vi "I(V)_K6221-K2182a_PK.vi"() -> ()   [LabVIEW 2016]
uses:
  Labview Drivers/Keithley 622x LV 2009/Keithley 622x.lvlib
panel:
  out "Resistance (ohm)":dbl=inf format="%#_13g"
  out "Time (s)":dbl=183.05660459992941 format="%#_13g"
  in  "Total number of I-V loops":i32=1
  in  "Numeric Average":i32=1
  in  "wait (ms)":u32=50
  out "Iset (A)":dbl
  out "Vmeas (V)":dbl=5.23101808e-07
  in  "Folder":path=path "D:/Pranava/Data/PtTe2/31-05-2022/001/Round8_IP/after warmup"
  in  "Set Compliance voltage (V)":dbl=2.0 min=0.0 step=0.1 format="%_3f"
  out "I vs V":cluster{dbl, "Field Reading":dbl}[](graph)=[{0.0, "Field Reading"=-1.0306718e-07}, {1e-07, "Field Reading"=-6.16332151e-08}, {2e-07, "Field Reading"=7.87243392e-08}, {3e-07, "Field Reading"=1.57966796e-07}, {4e-07, "Field Reading"=4.14402344e-09}, {5e-07, "Field Reading"=-1.72986197e-07}, {6e-07, "Field Reading"=6.26695055e-08}, {7e-07, "Field Reading"=8.13147919e-08}, {8e-07, "Field Reading"=1.95776133e-07}, {9e-07, "Field Reading"=1.06693098e-07}, {1e-06, "Field Reading"=1.80756319e-07}, {1.1e-06, "Field Reading"=-4.14238014e-09}, {1.2e-06, "Field Reading"=-1.20157502e-07}, {1.3e-06, "Field Reading"=1.29491334e-08}, {1.4e-06, "Field Reading"=1.86453892e-07}, {1.5e-06, "Field Reading"=9.68529269e-08}, {1.6e-06, "Field Reading"=-7.61339067e-08}, {1.7e-06, "Field Reading"=2.95227222e-08}, {1.8e-06, "Field Reading"=-1.09281084e-07}, {1.9e-06, "Field Reading"=4.60959452e-08}, {2e-06, "Field Reading"=2.19600694e-07}, {2.1e-06, "Field Reading"=-3.47002959e-08}, {2.2e-06, "Field Reading"=-7.2502909e-09}, {2.3e-06, "Field Reading"=-1.22747482e-07}, {2.4e-06, "Field Reading"=1.51234644e-07}, {2.5e-06, "Field Reading"=2.13903523e-07}, {2.6e-06, "Field Reading"=-1.10320173e-07}, {2.7e-06, "Field Reading"=-9.78899879e-08}, {2.8e-06, "Field Reading"=3.57345042e-08}, {2.9e-06, "Field Reading"=1.22745801e-07}, {3e-06, "Field Reading"=1.53821265e-07}, {3.1e-06, "Field Reading"=5.17696534e-09}, {3.2e-06, "Field Reading"=1.97326913e-07}, {3.3e-06, "Field Reading"=-6.94037265e-08}, {3.4e-06, "Field Reading"=-1.25857489e-07}, {3.5e-06, "Field Reading"=1.51750002e-07}, {3.6e-06, "Field Reading"=2.50673566e-07}, {3.7e-06, "Field Reading"=7.6133036e-08}, {3.8e-06, "Field Reading"=-1.42948994e-07}, {3.9e-06, "Field Reading"=7.76701235e-09}, {4e-06, "Field Reading"=1.305151e-07}, {4.1e-06, "Field Reading"=1.63142241e-07}, {4.2e-06, "Field Reading"=3.10364491e-09}, {4.3e-06, "Field Reading"=-6.21899174e-09}, {4.4e-06, "Field Reading"=3.21074034e-08}, {4.5e-06, "Field Reading"=6.72911471e-09}, {4.6e-06, "Field Reading"=2.5374388e-08}, {4.7e-06, "Field Reading"=7.04337985e-08}, {4.8e-06, "Field Reading"=-8.80770635e-09}, {4.9e-06, "Field Reading"=-1.24331767e-08}, {5e-06, "Field Reading"=-1.79722736e-07}, {5.1e-06, "Field Reading"=7.66498082e-08}, {5.2e-06, "Field Reading"=1.81270523e-07}, {5.3e-06, "Field Reading"=1.70885102e-08}, {5.4e-06, "Field Reading"=-5.54208961e-08}, {5.5e-06, "Field Reading"=-5.38662375e-08}, {5.6e-06, "Field Reading"=1.13922372e-08}, {5.7e-06, "Field Reading"=9.58139147e-08}, {5.8e-06, "Field Reading"=1.48124279e-07}, {5.9e-06, "Field Reading"=1.15495042e-07}, {6e-06, "Field Reading"=-1.23786032e-07}, {6.1e-06, "Field Reading"=2.2786574e-08}, {6.2e-06, "Field Reading"=1.53821448e-07}, {6.3e-06, "Field Reading"=9.21858153e-08}, {6.4e-06, "Field Reading"=1.43978235e-07}, {6.5e-06, "Field Reading"=1.76047313e-08}, {6.6e-06, "Field Reading"=1.2118957e-07}, {6.7e-06, "Field Reading"=5.48952733e-08}, {6.8e-06, "Field Reading"=2.49634771e-07}, {6.9e-06, "Field Reading"=1.08241465e-07}, {7e-06, "Field Reading"=1.1445703e-07}, {7.1e-06, "Field Reading"=-4.29919365e-08}, {7.2e-06, "Field Reading"=-6.73724028e-09}, {7.3e-06, "Field Reading"=-1.37772071e-07}, {7.4e-06, "Field Reading"=5.59315918e-08}, {7.5e-06, "Field Reading"=-5.18346759e-09}, {7.6e-06, "Field Reading"=1.19080321e-08}, {7.7e-06, "Field Reading"=9.37431805e-08}, {7.8e-06, "Field Reading"=-3.10869695e-09}, {7.9e-06, "Field Reading"=1.55894118e-07}, {8e-06, "Field Reading"=1.97846001e-07}, {8.1e-06, "Field Reading"=-7.2510577e-08}, {8.2e-06, "Field Reading"=2.01979046e-08}, {8.3e-06, "Field Reading"=1.89041284e-07}, {8.4e-06, "Field Reading"=2.00953547e-07}, {8.5e-06, "Field Reading"=1.25336495e-07}, {8.6e-06, "Field Reading"=-2.95229225e-08}, {8.7e-06, "Field Reading"=-3.21125449e-08}, {8.8e-06, "Field Reading"=1.46053473e-07}, {8.9e-06, "Field Reading"=4.81657483e-08}, {9e-06, "Field Reading"=3.2629119e-07}, {9.1e-06, "Field Reading"=-2.22719799e-08}, {9.2e-06, "Field Reading"=-3.36631723e-08}, {9.3e-06, "Field Reading"=4.14533263e-09}, {9.4e-06, "Field Reading"=1.62630298e-07}, {9.5e-06, "Field Reading"=2.13904846e-07}, {9.6e-06, "Field Reading"=1.09284052e-07}, {9.7e-06, "Field Reading"=7.19934716e-08}, {9.8e-06, "Field Reading"=3.05594936e-08}, {9.9e-06, "Field Reading"=3.41826524e-08}, {1e-05, "Field Reading"=2.29958129e-07}, {1.01e-05, "Field Reading"=1.10835484e-07}, {1.02e-05, "Field Reading"=5.74892568e-08}, {1.03e-05, "Field Reading"=-1.50198484e-07}, {1.04e-05, "Field Reading"=1.27926994e-07}, {1.05e-05, "Field Reading"=6.21505776e-08}, {1.06e-05, "Field Reading"=2.04579826e-07}, {1.07e-05, "Field Reading"=7.97590954e-08}, {1.08e-05, "Field Reading"=8.75279624e-08}, {1.09e-05, "Field Reading"=1.05137394e-07}, {1.1e-05, "Field Reading"=9.83929215e-09}, {1.11e-05, "Field Reading"=2.01471345e-07}, {1.12e-05, "Field Reading"=1.77128895e-07}, {1.13e-05, "Field Reading"=3.625344e-08}, {1.14e-05, "Field Reading"=-7.92397757e-08}, {1.15e-05, "Field Reading"=1.2585844e-07}, {1.16e-05, "Field Reading"=1.28965989e-07}, {1.17e-05, "Field Reading"=2.76056628e-07}, {1.18e-05, "Field Reading"=1.09284847e-07}, {1.19e-05, "Field Reading"=-1.65708764e-08}, {1.2e-05, "Field Reading"=7.87272845e-08}, {1.21e-05, "Field Reading"=1.05140243e-07}, {1.22e-05, "Field Reading"=2.38246889e-07}, {1.23e-05, "Field Reading"=1.02032695e-07}, {1.24e-05, "Field Reading"=5.80090957e-08}, {1.25e-05, "Field Reading"=1.11355339e-07}, {1.26e-05, "Field Reading"=1.65737432e-07}, {1.27e-05, "Field Reading"=1.9422329e-07}, {1.28e-05, "Field Reading"=2.24780847e-07}, {1.29e-05, "Field Reading"=1.08819028e-08}, {1.3e-05, "Field Reading"=1.2327163e-07}, {1.31e-05, "Field Reading"=7.45866788e-08}, {1.32e-05, "Field Reading"=2.26607776e-05}, {1.33e-05, "Field Reading"=2.30844403e-05}, {1.34e-05, "Field Reading"=2.30253968e-05}, {1.35e-05, "Field Reading"=2.31046393e-05}, {1.36e-05, "Field Reading"=2.33547805e-05}, {1.37e-05, "Field Reading"=2.36748579e-05}, {1.38e-05, "Field Reading"=2.39084419e-05}, {1.39e-05, "Field Reading"=2.39172467e-05}, {1.4e-05, "Field Reading"=2.41093967e-05}, {1.41e-05, "Field Reading"=2.42000335e-05}, {1.42e-05, "Field Reading"=2.44129006e-05}, {1.43e-05, "Field Reading"=2.46739283e-05}, {1.44e-05, "Field Reading"=2.49126915e-05}, {1.45e-05, "Field Reading"=2.50665151e-05}, {1.46e-05, "Field Reading"=2.49173528e-05}, {1.47e-05, "Field Reading"=2.53726085e-05}, {1.48e-05, "Field Reading"=2.56072284e-05}, {1.49e-05, "Field Reading"=2.57211718e-05}, {1.5e-05, "Field Reading"=2.58874256e-05}, {1.51e-05, "Field Reading"=2.59397274e-05}, {1.52e-05, "Field Reading"=2.62603227e-05}, {1.53e-05, "Field Reading"=2.64281302e-05}, {1.54e-05, "Field Reading"=2.65425915e-05}, {1.55e-05, "Field Reading"=2.69118716e-05}, {1.56e-05, "Field Reading"=2.69351782e-05}, {1.57e-05, "Field Reading"=2.69346603e-05}, {1.58e-05, "Field Reading"=2.71889769e-05}, {1.59e-05, "Field Reading"=2.76551091e-05}, {1.6e-05, "Field Reading"=2.7724511e-05}, {1.61e-05, "Field Reading"=2.77509251e-05}, {1.62e-05, "Field Reading"=2.79042308e-05}, {1.63e-05, "Field Reading"=2.81564602e-05}, {1.64e-05, "Field Reading"=2.83128734e-05}, {1.65e-05, "Field Reading"=2.85402591e-05}, {1.66e-05, "Field Reading"=2.878213e-05}, {1.67e-05, "Field Reading"=2.86754375e-05}, {1.68e-05, "Field Reading"=2.90255548e-05}, {1.69e-05, "Field Reading"=2.92524059e-05}, {1.7e-05, "Field Reading"=2.948599e-05}, {1.71e-05, "Field Reading"=2.95517665e-05}, {1.72e-05, "Field Reading"=2.96398137e-05}, {1.73e-05, "Field Reading"=2.98386812e-05}, {1.74e-05, "Field Reading"=2.99769671e-05}, {1.75e-05, "Field Reading"=3.02333399e-05}, {1.76e-05, "Field Reading"=3.06248909e-05}, {1.77e-05, "Field Reading"=3.07186353e-05}, {1.78e-05, "Field Reading"=3.0720707e-05}, {1.79e-05, "Field Reading"=3.07781966e-05}, {1.8e-05, "Field Reading"=3.11676923e-05}, {1.81e-05, "Field Reading"=3.14023123e-05}, {1.82e-05, "Field Reading"=3.14753397e-05}, {1.83e-05, "Field Reading"=3.14453001e-05}, {1.84e-05, "Field Reading"=3.17555371e-05}, {1.85e-05, "Field Reading"=3.203936e-05}, {1.86e-05, "Field Reading"=3.2266729e-05}, {1.87e-05, "Field Reading"=3.2533957e-05}, {1.88e-05, "Field Reading"=3.24930409e-05}, {1.89e-05, "Field Reading"=3.25805702e-05}, {1.9e-05, "Field Reading"=3.27084976e-05}, {1.91e-05, "Field Reading"=3.31010845e-05}, {1.92e-05, "Field Reading"=3.33186128e-05}, {1.93e-05, "Field Reading"=3.33092902e-05}, {1.94e-05, "Field Reading"=3.35133525e-05}, {1.95e-05, "Field Reading"=3.36200314e-05}, {1.96e-05, "Field Reading"=3.38396313e-05}, {1.97e-05, "Field Reading"=3.42684728e-05}, {1.98e-05, "Field Reading"=3.43093888e-05}, {1.99e-05, "Field Reading"=3.4376719e-05}, {2e-05, "Field Reading"=3.4630502e-05}, {2.01e-05, "Field Reading"=3.48371538e-05}, {2.02e-05, "Field Reading"=3.50759123e-05}, {2.03e-05, "Field Reading"=3.52696161e-05}, {2.04e-05, "Field Reading"=3.52986198e-05}, {2.05e-05, "Field Reading"=3.54146349e-05}, {2.06e-05, "Field Reading"=3.56922424e-05}, {2.07e-05, "Field Reading"=3.58439942e-05}, {2.08e-05, "Field Reading"=3.61733941e-05}, {2.09e-05, "Field Reading"=3.62407028e-05}, {2.1e-05, "Field Reading"=3.63385905e-05}, {2.11e-05, "Field Reading"=3.65343658e-05}, {2.12e-05, "Field Reading"=3.68093835e-05}, {2.13e-05, "Field Reading"=3.70973494e-05}, {2.14e-05, "Field Reading"=3.70709352e-05}, {2.15e-05, "Field Reading"=3.72884634e-05}, {2.16e-05, "Field Reading"=3.74443585e-05}, {2.17e-05, "Field Reading"=3.75831529e-05}, {2.18e-05, "Field Reading"=3.7787215e-05}, {2.19e-05, "Field Reading"=3.808036e-05}, {2.2e-05, "Field Reading"=3.80984874e-05}, {2.21e-05, "Field Reading"=3.8141475e-05}, {2.22e-05, "Field Reading"=3.84734643e-05}, {2.23e-05, "Field Reading"=3.87127452e-05}, {2.24e-05, "Field Reading"=3.88867762e-05}, {2.25e-05, "Field Reading"=3.90576911e-05}, {2.26e-05, "Field Reading"=3.91959769e-05}, {2.27e-05, "Field Reading"=3.9318207e-05}, {2.28e-05, "Field Reading"=3.95512728e-05}, {2.29e-05, "Field Reading"=3.98946565e-05}, {2.3e-05, "Field Reading"=4.00065281e-05}, {2.31e-05, "Field Reading"=4.00277984e-05}, {2.32e-05, "Field Reading"=4.02308248e-05}, {2.33e-05, "Field Reading"=4.04452456e-05}, {2.34e-05, "Field Reading"=4.06151248e-05}, {2.35e-05, "Field Reading"=4.08015776e-05}, {2.36e-05, "Field Reading"=4.10191059e-05}, {2.37e-05, "Field Reading"=4.11428899e-05}, {2.38e-05, "Field Reading"=4.12573512e-05}, {2.39e-05, "Field Reading"=4.1494075e-05}, {2.4e-05, "Field Reading"=4.17799696e-05}, {2.41e-05, "Field Reading"=4.19229168e-05}, {2.42e-05, "Field Reading"=4.19032357e-05}, {2.43e-05, "Field Reading"=4.21290509e-05}, {2.44e-05, "Field Reading"=4.22953048e-05}, {2.45e-05, "Field Reading"=4.26832305e-05}, {2.46e-05, "Field Reading"=4.28903968e-05}, {2.47e-05, "Field Reading"=4.29478865e-05}, {2.48e-05, "Field Reading"=4.30939413e-05}, {2.49e-05, "Field Reading"=4.32783225e-05}, {2.5e-05, "Field Reading"=4.35756113e-05}, {2.51e-05, "Field Reading"=4.37413473e-05}, {2.52e-05, "Field Reading"=4.394282e-05}, {2.53e-05, "Field Reading"=4.40370823e-05}, {2.54e-05, "Field Reading"=4.41116635e-05}, {2.55e-05, "Field Reading"=4.42986344e-05}, {2.56e-05, "Field Reading"=4.46016204e-05}, {2.57e-05, "Field Reading"=4.49289489e-05}, {2.58e-05, "Field Reading"=4.4907196e-05}, {2.59e-05, "Field Reading"=4.49828131e-05}, {2.6e-05, "Field Reading"=4.51438877e-05}, {2.61e-05, "Field Reading"=4.53893525e-05}, {2.62e-05, "Field Reading"=4.57192705e-05}, {2.63e-05, "Field Reading"=4.58549667e-05}, {2.64e-05, "Field Reading"=4.59787506e-05}, {2.65e-05, "Field Reading"=4.61569167e-05}, {2.66e-05, "Field Reading"=4.6195761e-05}, {2.67e-05, "Field Reading"=4.65381091e-05}, {2.68e-05, "Field Reading"=4.68421046e-05}, {2.69e-05, "Field Reading"=4.69166857e-05}, {2.7e-05, "Field Reading"=4.69291159e-05}, {2.71e-05, "Field Reading"=4.70637762e-05}, {2.72e-05, "Field Reading"=4.74589524e-05}, {2.73e-05, "Field Reading"=4.76852853e-05}, {2.74e-05, "Field Reading"=4.7755723e-05}, {2.75e-05, "Field Reading"=4.79189044e-05}, {2.76e-05, "Field Reading"=4.80960347e-05}, {2.77e-05, "Field Reading"=4.8176313e-05}, {2.78e-05, "Field Reading"=4.85476649e-05}, {2.79e-05, "Field Reading"=4.87708904e-05}, {2.8e-05, "Field Reading"=4.86621262e-05}, {2.81e-05, "Field Reading"=4.89531998e-05}, {2.82e-05, "Field Reading"=4.91298121e-05}, {2.83e-05, "Field Reading"=4.93898453e-05}, {2.84e-05, "Field Reading"=4.9613071e-05}, {2.85e-05, "Field Reading"=4.97399626e-05}, {2.86e-05, "Field Reading"=4.98943042e-05}, {2.87e-05, "Field Reading"=4.98109183e-05}, {2.88e-05, "Field Reading"=5.01926289e-05}, {2.89e-05, "Field Reading"=5.05764113e-05}, {2.9e-05, "Field Reading"=5.06804975e-05}, {2.91e-05, "Field Reading"=5.06680673e-05}, {2.92e-05, "Field Reading"=5.07587041e-05}, {2.93e-05, "Field Reading"=5.11942789e-05}, {2.94e-05, "Field Reading"=5.126886e-05}, {2.95e-05, "Field Reading"=5.15138384e-05}, {2.96e-05, "Field Reading"=5.16236385e-05}, {2.97e-05, "Field Reading"=5.17816017e-05}, {2.98e-05, "Field Reading"=5.19965405e-05}, {2.99e-05, "Field Reading"=5.21840292e-05}, {3e-05, "Field Reading"=5.24512784e-05}, {3e-05, "Field Reading"=5.23492472e-05}, {2.99e-05, "Field Reading"=5.22622359e-05}, {2.98e-05, "Field Reading"=5.19255848e-05}, {2.97e-05, "Field Reading"=5.18157848e-05}, {2.96e-05, "Field Reading"=5.18442655e-05}, {2.95e-05, "Field Reading"=5.17018363e-05}, {2.94e-05, "Field Reading"=5.13310022e-05}, {2.93e-05, "Field Reading"=5.10901672e-05}, {2.92e-05, "Field Reading"=5.09461842e-05}, {2.91e-05, "Field Reading"=5.08710851e-05}, {2.9e-05, "Field Reading"=5.07504086e-05}, {2.89e-05, "Field Reading"=5.04069981e-05}, {2.88e-05, "Field Reading"=5.03842094e-05}, {2.87e-05, "Field Reading"=5.00076783e-05}, {2.86e-05, "Field Reading"=4.98393529e-05}, {2.85e-05, "Field Reading"=4.98072416e-05}, {2.84e-05, "Field Reading"=4.97787557e-05}, {2.83e-05, "Field Reading"=4.92551341e-05}, {2.82e-05, "Field Reading"=4.91329288e-05}, {2.81e-05, "Field Reading"=4.90909769e-05}, {2.8e-05, "Field Reading"=4.89148825e-05}, {2.79e-05, "Field Reading"=4.88750023e-05}, {2.78e-05, "Field Reading"=4.85186701e-05}, {2.77e-05, "Field Reading"=4.84611805e-05}, {2.76e-05, "Field Reading"=4.79670804e-05}, {2.75e-05, "Field Reading"=4.794222e-05}, {2.74e-05, "Field Reading"=4.79997168e-05}, {2.73e-05, "Field Reading"=4.7894578e-05}, {2.72e-05, "Field Reading"=4.74450194e-05}, {2.71e-05, "Field Reading"=4.71798419e-05}, {2.7e-05, "Field Reading"=4.71342645e-05}, {2.69e-05, "Field Reading"=4.70327513e-05}, {2.68e-05, "Field Reading"=4.68369757e-05}, {2.67e-05, "Field Reading"=4.66453199e-05}, {2.66e-05, "Field Reading"=4.64552416e-05}, {2.65e-05, "Field Reading"=4.61289491e-05}, {2.64e-05, "Field Reading"=4.60574756e-05}, {2.63e-05, "Field Reading"=4.59326557e-05}, {2.62e-05, "Field Reading"=4.57897086e-05}, {2.61e-05, "Field Reading"=4.55690727e-05}, {2.6e-05, "Field Reading"=4.53670553e-05}, {2.59e-05, "Field Reading"=4.51086111e-05}, {2.58e-05, "Field Reading"=4.51402045e-05}, {2.57e-05, "Field Reading"=4.5013831e-05}, {2.56e-05, "Field Reading"=4.45886152e-05}, {2.55e-05, "Field Reading"=4.43975011e-05}, {2.54e-05, "Field Reading"=4.42659484e-05}, {2.53e-05, "Field Reading"=4.42783786e-05}, {2.52e-05, "Field Reading"=4.4098133e-05}, {2.51e-05, "Field Reading"=4.38241511e-05}, {2.5e-05, "Field Reading"=4.36066229e-05}, {2.49e-05, "Field Reading"=4.35335956e-05}, {2.48e-05, "Field Reading"=4.31845148e-05}, {2.47e-05, "Field Reading"=4.3292243e-05}, {2.46e-05, "Field Reading"=4.31876223e-05}, {2.45e-05, "Field Reading"=4.27178684e-05}, {2.44e-05, "Field Reading"=4.25132884e-05}, {2.43e-05, "Field Reading"=4.23843252e-05}, {2.42e-05, "Field Reading"=4.23439272e-05}, {2.41e-05, "Field Reading"=4.22191074e-05}, {2.4e-05, "Field Reading"=4.20766783e-05}, {2.39e-05, "Field Reading"=4.17011832e-05}, {2.38e-05, "Field Reading"=4.15660192e-05}, {2.37e-05, "Field Reading"=4.13101646e-05}, {2.36e-05, "Field Reading"=4.12019184e-05}, {2.35e-05, "Field Reading"=4.12506033e-05}, {2.34e-05, "Field Reading"=4.08316025e-05}, {2.33e-05, "Field Reading"=4.06140743e-05}, {2.32e-05, "Field Reading"=4.05224017e-05}, {2.31e-05, "Field Reading"=4.03825621e-05}, {2.3e-05, "Field Reading"=4.02712359e-05}, {2.29e-05, "Field Reading"=4.00718349e-05}, {2.28e-05, "Field Reading"=3.96419574e-05}, {2.27e-05, "Field Reading"=3.95616791e-05}, {2.26e-05, "Field Reading"=3.954148e-05}, {2.25e-05, "Field Reading"=3.93596885e-05}, {2.24e-05, "Field Reading"=3.92970196e-05}, {2.23e-05, "Field Reading"=3.89966273e-05}, {2.22e-05, "Field Reading"=3.87247169e-05}, {2.21e-05, "Field Reading"=3.85626064e-05}, {2.2e-05, "Field Reading"=3.85646781e-05}, {2.19e-05, "Field Reading"=3.83637233e-05}, {2.18e-05, "Field Reading"=3.81353185e-05}, {2.17e-05, "Field Reading"=3.7795042e-05}, {2.16e-05, "Field Reading"=3.77416642e-05}, {2.15e-05, "Field Reading"=3.75935378e-05}, {2.14e-05, "Field Reading"=3.74614671e-05}, {2.13e-05, "Field Reading"=3.72662096e-05}, {2.12e-05, "Field Reading"=3.72004332e-05}, {2.11e-05, "Field Reading"=3.67658947e-05}, {2.1e-05, "Field Reading"=3.67462136e-05}, {2.09e-05, "Field Reading"=3.66597202e-05}, {2.08e-05, "Field Reading"=3.65121165e-05}, {2.07e-05, "Field Reading"=3.61992902e-05}, {2.06e-05, "Field Reading"=3.60371798e-05}, {2.05e-05, "Field Reading"=3.58382969e-05}, {2.04e-05, "Field Reading"=3.58035959e-05}, {2.03e-05, "Field Reading"=3.56699714e-05}, {2.02e-05, "Field Reading"=3.53680215e-05}, {2.01e-05, "Field Reading"=3.5284114e-05}, {2e-05, "Field Reading"=3.49588575e-05}, {1.99e-05, "Field Reading"=3.48128029e-05}, {1.98e-05, "Field Reading"=3.46719275e-05}, {1.97e-05, "Field Reading"=3.46382624e-05}, {1.96e-05, "Field Reading"=3.44782238e-05}, {1.95e-05, "Field Reading"=3.40566333e-05}, {1.94e-05, "Field Reading"=3.39380163e-05}, {1.93e-05, "Field Reading"=3.3864471e-05}, {1.92e-05, "Field Reading"=3.37702088e-05}, {1.91e-05, "Field Reading"=3.33993751e-05}, {1.9e-05, "Field Reading"=3.33009695e-05}, {1.89e-05, "Field Reading"=3.31865083e-05}, {1.88e-05, "Field Reading"=3.28483038e-05}, {1.87e-05, "Field Reading"=3.2840017e-05}, {1.86e-05, "Field Reading"=3.2770645e-05}, {1.85e-05, "Field Reading"=3.24774997e-05}, {1.84e-05, "Field Reading"=3.21273827e-05}, {1.83e-05, "Field Reading"=3.198081e-05}, {1.82e-05, "Field Reading"=3.19005317e-05}, {1.81e-05, "Field Reading"=3.19274638e-05}, {1.8e-05, "Field Reading"=3.16332826e-05}, {1.79e-05, "Field Reading"=3.13919284e-05}, {1.78e-05, "Field Reading"=3.12945586e-05}, {1.77e-05, "Field Reading"=3.1037668e-05}, {1.76e-05, "Field Reading"=3.0982768e-05}, {1.75e-05, "Field Reading"=3.07522915e-05}, {1.74e-05, "Field Reading"=3.05114566e-05}, {1.73e-05, "Field Reading"=3.03555613e-05}, {1.72e-05, "Field Reading"=2.9926711e-05}, {1.71e-05, "Field Reading"=2.99919695e-05}, {1.7e-05, "Field Reading"=2.98562733e-05}, {1.69e-05, "Field Reading"=2.97961941e-05}, {1.68e-05, "Field Reading"=2.94077507e-05}, {1.67e-05, "Field Reading"=2.92373536e-05}, {1.66e-05, "Field Reading"=2.89794272e-05}, {1.65e-05, "Field Reading"=2.90410602e-05}, {1.64e-05, "Field Reading"=2.9025534e-05}, {1.63e-05, "Field Reading"=2.8613266e-05}, {1.62e-05, "Field Reading"=2.8304065e-05}, {1.61e-05, "Field Reading"=2.81833885e-05}, {1.6e-05, "Field Reading"=2.82476112e-05}, {1.59e-05, "Field Reading"=2.79477328e-05}, {1.58e-05, "Field Reading"=2.77835507e-05}, {1.57e-05, "Field Reading"=2.76204056e-05}, {1.56e-05, "Field Reading"=2.74230763e-05}, {1.55e-05, "Field Reading"=2.71273413e-05}, {1.54e-05, "Field Reading"=2.70154696e-05}, {1.53e-05, "Field Reading"=2.69175818e-05}, {1.52e-05, "Field Reading"=2.67647941e-05}, {1.51e-05, "Field Reading"=2.65156723e-05}, {1.5e-05, "Field Reading"=2.61707402e-05}, {1.49e-05, "Field Reading"=2.59412995e-05}, {1.48e-05, "Field Reading"=2.62018157e-05}, {1.47e-05, "Field Reading"=2.58382325e-05}, {1.46e-05, "Field Reading"=2.55549277e-05}, {1.45e-05, "Field Reading"=2.53472399e-05}, {1.44e-05, "Field Reading"=2.51789143e-05}, {1.43e-05, "Field Reading"=2.52317427e-05}, {1.42e-05, "Field Reading"=2.49158009e-05}, {1.41e-05, "Field Reading"=2.4860383e-05}, {1.4e-05, "Field Reading"=2.4564648e-05}, {1.39e-05, "Field Reading"=2.44734933e-05}, {1.38e-05, "Field Reading"=2.4090747e-05}, {1.37e-05, "Field Reading"=2.41896706e-05}, {1.36e-05, "Field Reading"=2.40135762e-05}, {1.35e-05, "Field Reading"=2.36494645e-05}, {1.34e-05, "Field Reading"=2.34490277e-05}, {1.33e-05, "Field Reading"=2.34132909e-05}, {1.32e-05, "Field Reading"=2.32630928e-05}, {1.31e-05, "Field Reading"=2.30554051e-05}, {1.3e-05, "Field Reading"=2.2857558e-05}, {1.29e-05, "Field Reading"=2.26534958e-05}, {1.28e-05, "Field Reading"=2.24659978e-05}, {1.27e-05, "Field Reading"=2.21987489e-05}, {1.26e-05, "Field Reading"=2.21935697e-05}, {1.25e-05, "Field Reading"=2.21143273e-05}, {1.24e-05, "Field Reading"=2.17611029e-05}, {1.23e-05, "Field Reading"=2.14622606e-05}, {1.22e-05, "Field Reading"=2.12483579e-05}, {1.21e-05, "Field Reading"=2.13529786e-05}, {1.2e-05, "Field Reading"=2.11416515e-05}, {1.19e-05, "Field Reading"=2.08101801e-05}, {1.18e-05, "Field Reading"=2.06154407e-05}, {1.17e-05, "Field Reading"=2.04750833e-05}, {1.16e-05, "Field Reading"=2.03026146e-05}, {1.15e-05, "Field Reading"=2.02016194e-05}, {1.14e-05, "Field Reading"=2.00322583e-05}, {1.13e-05, "Field Reading"=1.98173324e-05}, {1.12e-05, "Field Reading"=1.95884099e-05}, {1.11e-05, "Field Reading"=1.93770968e-05}, {1.1e-05, "Field Reading"=1.94936298e-05}, {1.09e-05, "Field Reading"=1.92268988e-05}, {1.08e-05, "Field Reading"=1.8910965e-05}, {1.07e-05, "Field Reading"=1.86789349e-05}, {1.06e-05, "Field Reading"=1.83878552e-05}, {1.05e-05, "Field Reading"=1.84510419e-05}, {1.04e-05, "Field Reading"=1.81604865e-05}, {1.03e-05, "Field Reading"=1.80449894e-05}, {1.02e-05, "Field Reading"=1.78657877e-05}, {1.01e-05, "Field Reading"=1.75462285e-05}, {1e-05, "Field Reading"=1.73349154e-05}, {9.9e-06, "Field Reading"=1.73618475e-05}, {9.8e-06, "Field Reading"=1.71360338e-05}, {9.7e-06, "Field Reading"=1.6854801e-05}, {9.6e-06, "Field Reading"=1.65616559e-05}, {9.5e-06, "Field Reading"=1.63736494e-05}, {9.4e-06, "Field Reading"=1.64119758e-05}, {9.3e-06, "Field Reading"=1.62643674e-05}, {9.2e-06, "Field Reading"=1.5946362e-05}, {9.1e-06, "Field Reading"=1.58489938e-05}, {9e-06, "Field Reading"=1.54393158e-05}, {8.9e-06, "Field Reading"=1.53378026e-05}, {8.8e-06, "Field Reading"=1.51435811e-05}, {8.7e-06, "Field Reading"=1.51182028e-05}, {8.6e-06, "Field Reading"=1.48561331e-05}, {8.5e-06, "Field Reading"=1.45370918e-05}, {8.4e-06, "Field Reading"=1.44039845e-05}, {8.3e-06, "Field Reading"=1.44112355e-05}, {8.2e-06, "Field Reading"=1.41952611e-05}, {8.1e-06, "Field Reading"=1.39326736e-05}, {8e-06, "Field Reading"=1.36125964e-05}, {7.9e-06, "Field Reading"=1.34535937e-05}, {7.8e-06, "Field Reading"=1.32925193e-05}, {7.7e-06, "Field Reading"=1.29838365e-05}, {7.6e-06, "Field Reading"=1.29879856e-05}, {7.5e-06, "Field Reading"=1.27683857e-05}, {7.4e-06, "Field Reading"=1.23126123e-05}, {7.3e-06, "Field Reading"=1.21898643e-05}, {7.2e-06, "Field Reading"=1.2143769e-05}, {7.1e-06, "Field Reading"=1.20645266e-05}, {7e-06, "Field Reading"=1.17636125e-05}, {6.9e-06, "Field Reading"=1.15088055e-05}, {6.8e-06, "Field Reading"=1.13648224e-05}, {6.7e-06, "Field Reading"=1.12493252e-05}, {6.6e-06, "Field Reading"=1.12835082e-05}, {6.5e-06, "Field Reading"=1.10235101e-05}, {6.4e-06, "Field Reading"=1.0789926e-05}, {6.3e-06, "Field Reading"=1.03471005e-05}, {6.2e-06, "Field Reading"=9.88614346e-06}, {6.1e-06, "Field Reading"=9.84988874e-06}, {6e-06, "Field Reading"=9.49977175e-06}, {5.9e-06, "Field Reading"=9.02638873e-06}, {5.8e-06, "Field Reading"=8.74670948e-06}, {5.7e-06, "Field Reading"=8.36137362e-06}, {5.6e-06, "Field Reading"=8.34894343e-06}, {5.5e-06, "Field Reading"=7.80615851e-06}, {5.4e-06, "Field Reading"=4.17187494e-06}, {5.3e-06, "Field Reading"=7.10587483e-07}, {5.2e-06, "Field Reading"=4.5784047e-07}, {5.1e-06, "Field Reading"=5.61425311e-07}, {5e-06, "Field Reading"=6.74850713e-07}, {4.9e-06, "Field Reading"=7.08515786e-07}, {4.8e-06, "Field Reading"=5.56763993e-07}, {4.7e-06, "Field Reading"=4.38163618e-07}, {4.6e-06, "Field Reading"=7.12145693e-07}, {4.5e-06, "Field Reading"=6.80034372e-07}, {4.4e-06, "Field Reading"=7.17324938e-07}, {4.3e-06, "Field Reading"=6.67086259e-07}, {4.2e-06, "Field Reading"=5.30354184e-07}, {4.1e-06, "Field Reading"=4.44896637e-07}, {4e-06, "Field Reading"=5.80068727e-07}, {3.9e-06, "Field Reading"=7.13693138e-07}, {3.8e-06, "Field Reading"=5.60905537e-07}, {3.7e-06, "Field Reading"=5.00826345e-07}, {3.6e-06, "Field Reading"=5.74889487e-07}, {3.5e-06, "Field Reading"=5.95088525e-07}, {3.4e-06, "Field Reading"=6.86243162e-07}, {3.3e-06, "Field Reading"=6.45845084e-07}, {3.2e-06, "Field Reading"=6.98152947e-07}, {3.1e-06, "Field Reading"=5.94050244e-07}, {3e-06, "Field Reading"=5.12736193e-07}, {2.9e-06, "Field Reading"=5.33453149e-07}, {2.8e-06, "Field Reading"=6.59826579e-07}, {2.7e-06, "Field Reading"=5.82655919e-07}, {2.6e-06, "Field Reading"=3.41303385e-07}, {2.5e-06, "Field Reading"=4.90989519e-07}, {2.4e-06, "Field Reading"=6.650121e-07}, {2.3e-06, "Field Reading"=7.24055475e-07}, {2.2e-06, "Field Reading"=6.0907627e-07}, {2.1e-06, "Field Reading"=5.87841372e-07}, {2e-06, "Field Reading"=6.03379102e-07}, {1.9e-06, "Field Reading"=5.5780176e-07}, {1.8e-06, "Field Reading"=5.03419671e-07}, {1.7e-06, "Field Reading"=6.94015831e-07}, {1.6e-06, "Field Reading"=6.28239439e-07}, {1.5e-06, "Field Reading"=5.62980971e-07}, {1.4e-06, "Field Reading"=3.75492358e-07}, {1.3e-06, "Field Reading"=6.20988498e-07}, {1.2e-06, "Field Reading"=6.69673386e-07}, {1.1e-06, "Field Reading"=7.23019594e-07}, {1e-06, "Field Reading"=4.88920827e-07}, {9e-07, "Field Reading"=5.12745357e-07}, {8e-07, "Field Reading"=4.75972712e-07}, {7e-07, "Field Reading"=6.18401969e-07}, {6e-07, "Field Reading"=5.57804795e-07}, {5e-07, "Field Reading"=6.72266125e-07}, {4e-07, "Field Reading"=5.50553851e-07}, {3e-07, "Field Reading"=3.9517723e-07}, {2e-07, "Field Reading"=5.36052729e-07}, {1e-07, "Field Reading"=6.39637654e-07}, {0.0, "Field Reading"=6.78482001e-07}, {-1e-07, "Field Reading"=3.96213079e-07}, {-2e-07, "Field Reading"=4.45415919e-07}, {-3e-07, "Field Reading"=5.31391407e-07}, {-4e-07, "Field Reading"=5.06008609e-07}, {-5e-07, "Field Reading"=6.54134958e-07}, {-6e-07, "Field Reading"=6.3393591e-07}, {-7e-07, "Field Reading"=5.51068023e-07}, {-8e-07, "Field Reading"=4.38678451e-07}, {-9e-07, "Field Reading"=4.92542578e-07}, {-1e-06, "Field Reading"=6.40151002e-07}, {-1.1e-06, "Field Reading"=5.59354812e-07}, {-1.2e-06, "Field Reading"=4.94612845e-07}, {-1.3e-06, "Field Reading"=4.15370444e-07}, {-1.4e-06, "Field Reading"=5.33975084e-07}, {-1.5e-06, "Field Reading"=5.31385463e-07}, {-1.6e-06, "Field Reading"=5.92500517e-07}, {-1.7e-06, "Field Reading"=5.62460914e-07}, {-1.8e-06, "Field Reading"=4.60947773e-07}, {-1.9e-06, "Field Reading"=4.6664634e-07}, {-2e-06, "Field Reading"=6.0545005e-07}, {-2.1e-06, "Field Reading"=6.66565117e-07}, {-2.2e-06, "Field Reading"=4.47483141e-07}, {-2.3e-06, "Field Reading"=4.24694472e-07}, {-2.4e-06, "Field Reading"=3.87403923e-07}, {-2.5e-06, "Field Reading"=6.42222675e-07}, {-2.6e-06, "Field Reading"=4.5577212e-07}, {-2.7e-06, "Field Reading"=4.7079193e-07}, {-2.8e-06, "Field Reading"=5.22584375e-07}, {-2.9e-06, "Field Reading"=3.66171189e-07}, {-3e-06, "Field Reading"=4.12266466e-07}, {-3.1e-06, "Field Reading"=4.73381552e-07}, {-3.2e-06, "Field Reading"=6.44814547e-07}, {-3.3e-06, "Field Reading"=5.81627763e-07}, {-3.4e-06, "Field Reading"=5.44342461e-07}, {-3.5e-06, "Field Reading"=3.44941395e-07}, {-3.6e-06, "Field Reading"=6.16851939e-07}, {-3.7e-06, "Field Reading"=5.03426398e-07}, {-3.8e-06, "Field Reading"=5.52111333e-07}, {-3.9e-06, "Field Reading"=5.27250941e-07}, {-4e-06, "Field Reading"=4.117537e-07}, {-4.1e-06, "Field Reading"=3.94141643e-07}, {-4.2e-06, "Field Reading"=6.15813392e-07}, {-4.3e-06, "Field Reading"=5.42268092e-07}, {-4.4e-06, "Field Reading"=5.13264312e-07}, {-4.5e-06, "Field Reading"=4.71312415e-07}, {-4.6e-06, "Field Reading"=3.70317109e-07}, {-4.7e-06, "Field Reading"=6.38602076e-07}, {-4.8e-06, "Field Reading"=5.58838451e-07}, {-4.9e-06, "Field Reading"=4.3660829e-07}, {-5e-06, "Field Reading"=5.28798835e-07}, {-5.1e-06, "Field Reading"=4.57843191e-07}, {-5.2e-06, "Field Reading"=5.13779027e-07}, {-5.3e-06, "Field Reading"=5.03420539e-07}, {-5.4e-06, "Field Reading"=5.52105434e-07}, {-5.5e-06, "Field Reading"=5.03938463e-07}, {-5.6e-06, "Field Reading"=4.3971918e-07}, {-5.7e-06, "Field Reading"=4.03464454e-07}, {-5.8e-06, "Field Reading"=5.41232414e-07}, {-5.9e-06, "Field Reading"=4.9410127e-07}, {-6e-06, "Field Reading"=5.619494e-07}, {-6.1e-06, "Field Reading"=4.5525692e-07}, {-6.2e-06, "Field Reading"=4.63543715e-07}, {-6.3e-06, "Field Reading"=4.69751015e-07}, {-6.4e-06, "Field Reading"=5.27240588e-07}, {-6.5e-06, "Field Reading"=6.66044241e-07}, {-6.6e-06, "Field Reading"=4.8943213e-07}, {-6.7e-06, "Field Reading"=5.96124491e-07}, {-6.8e-06, "Field Reading"=5.72299983e-07}, {-6.9e-06, "Field Reading"=4.72340636e-07}, {-7e-06, "Field Reading"=3.52184897e-07}, {-7.1e-06, "Field Reading"=4.41785798e-07}, {-7.2e-06, "Field Reading"=5.44334805e-07}, {-7.3e-06, "Field Reading"=6.07521567e-07}, {-7.4e-06, "Field Reading"=4.49036738e-07}, {-7.5e-06, "Field Reading"=3.3923679e-07}, {-7.6e-06, "Field Reading"=3.16966046e-07}, {-7.7e-06, "Field Reading"=4.84257305e-07}, {-7.8e-06, "Field Reading"=5.75929926e-07}, {-7.9e-06, "Field Reading"=4.58879009e-07}, {-8e-06, "Field Reading"=4.92026171e-07}, {-8.1e-06, "Field Reading"=3.93102609e-07}, {-8.2e-06, "Field Reading"=5.14814845e-07}, {-8.3e-06, "Field Reading"=4.56807312e-07}, {-8.4e-06, "Field Reading"=5.12742069e-07}, {-8.5e-06, "Field Reading"=6.33936362e-07}, {-8.6e-06, "Field Reading"=3.06090262e-07}, {-8.7e-06, "Field Reading"=2.72425181e-07}, {-8.8e-06, "Field Reading"=5.86805248e-07}, {-8.9e-06, "Field Reading"=5.79036383e-07}, {-9e-06, "Field Reading"=4.58877939e-07}, {-9.1e-06, "Field Reading"=4.13300598e-07}, {-9.2e-06, "Field Reading"=4.45933617e-07}, {-9.3e-06, "Field Reading"=4.39200597e-07}, {-9.4e-06, "Field Reading"=5.50036464e-07}, {-9.5e-06, "Field Reading"=5.06012872e-07}, {-9.6e-06, "Field Reading"=5.57287408e-07}, {-9.7e-06, "Field Reading"=4.80634566e-07}, {-9.8e-06, "Field Reading"=3.59958131e-07}, {-9.9e-06, "Field Reading"=5.83183472e-07}, {-1e-05, "Field Reading"=5.33980636e-07}, {-1.01e-05, "Field Reading"=4.5007685e-07}, {-1.02e-05, "Field Reading"=4.60435342e-07}, {-1.03e-05, "Field Reading"=4.21073073e-07}, {-1.04e-05, "Field Reading"=4.2521647e-07}, {-1.05e-05, "Field Reading"=4.43861755e-07}, {-1.06e-05, "Field Reading"=5.93540392e-07}, {-1.07e-05, "Field Reading"=4.46967763e-07}, {-1.08e-05, "Field Reading"=2.42905516e-07}, {-1.09e-05, "Field Reading"=5.13262097e-07}, {-1.1e-05, "Field Reading"=6.48958312e-07}, {-1.11e-05, "Field Reading"=5.77484733e-07}, {-1.12e-05, "Field Reading"=4.1433852e-07}, {-1.13e-05, "Field Reading"=6.09596051e-07}, {-1.14e-05, "Field Reading"=3.6047874e-07}, {-1.15e-05, "Field Reading"=6.01831704e-07}, {-1.16e-05, "Field Reading"=6.05457178e-07}, {-1.17e-05, "Field Reading"=6.17887373e-07}, {-1.18e-05, "Field Reading"=5.37609027e-07}, {-1.19e-05, "Field Reading"=2.89005116e-07}, {-1.2e-05, "Field Reading"=4.28326891e-07}, {-1.21e-05, "Field Reading"=7.01792144e-07}, {-1.22e-05, "Field Reading"=5.19482585e-07}, {-1.23e-05, "Field Reading"=4.35578754e-07}, {-1.24e-05, "Field Reading"=4.02949486e-07}, {-1.25e-05, "Field Reading"=4.24702331e-07}, {-1.26e-05, "Field Reading"=5.34502407e-07}, {-1.27e-05, "Field Reading"=6.57768529e-07}, {-1.28e-05, "Field Reading"=5.07569014e-07}, {-1.29e-05, "Field Reading"=5.43823749e-07}, {-1.3e-05, "Field Reading"=3.52709502e-07}, {-1.31e-05, "Field Reading"=5.37090727e-07}, {-1.32e-05, "Field Reading"=6.81591742e-07}, {-1.33e-05, "Field Reading"=4.91513345e-07}, {-1.34e-05, "Field Reading"=4.77011451e-07}, {-1.35e-05, "Field Reading"=3.87928388e-07}, {-1.36e-05, "Field Reading"=-2.27947894e-05}, {-1.37e-05, "Field Reading"=-2.28222392e-05}, {-1.38e-05, "Field Reading"=-2.29366998e-05}, {-1.39e-05, "Field Reading"=-2.32614363e-05}, {-1.4e-05, "Field Reading"=-2.34732661e-05}, {-1.41e-05, "Field Reading"=-2.37342984e-05}, {-1.42e-05, "Field Reading"=-2.36918288e-05}, {-1.43e-05, "Field Reading"=-2.37534459e-05}, {-1.44e-05, "Field Reading"=-2.42485781e-05}, {-1.45e-05, "Field Reading"=-2.44282966e-05}, {-1.46e-05, "Field Reading"=-2.45002876e-05}, {-1.47e-05, "Field Reading"=-2.46753448e-05}, {-1.48e-05, "Field Reading"=-2.48317569e-05}, {-1.49e-05, "Field Reading"=-2.49130704e-05}, {-1.5e-05, "Field Reading"=-2.51150617e-05}, {-1.51e-05, "Field Reading"=-2.5433065e-05}, {-1.52e-05, "Field Reading"=-2.5714296e-05}, {-1.53e-05, "Field Reading"=-2.56241778e-05}, {-1.54e-05, "Field Reading"=-2.56884e-05}, {-1.55e-05, "Field Reading"=-2.60074392e-05}, {-1.56e-05, "Field Reading"=-2.63078332e-05}, {-1.57e-05, "Field Reading"=-2.64481897e-05}, {-1.58e-05, "Field Reading"=-2.65522951e-05}, {-1.59e-05, "Field Reading"=-2.65771553e-05}, {-1.6e-05, "Field Reading"=-2.68568326e-05}, {-1.61e-05, "Field Reading"=-2.71080242e-05}, {-1.62e-05, "Field Reading"=-2.74146333e-05}, {-1.63e-05, "Field Reading"=-2.75684558e-05}, {-1.64e-05, "Field Reading"=-2.75829576e-05}, {-1.65e-05, "Field Reading"=-2.7660124e-05}, {-1.66e-05, "Field Reading"=-2.79553388e-05}, {-1.67e-05, "Field Reading"=-2.8097767e-05}, {-1.68e-05, "Field Reading"=-2.84225033e-05}, {-1.69e-05, "Field Reading"=-2.85043348e-05}, {-1.7e-05, "Field Reading"=-2.85499118e-05}, {-1.71e-05, "Field Reading"=-2.87555264e-05}, {-1.72e-05, "Field Reading"=-2.91284301e-05}, {-1.73e-05, "Field Reading"=-2.92278709e-05}, {-1.74e-05, "Field Reading"=-2.9318507e-05}, {-1.75e-05, "Field Reading"=-2.95220499e-05}, {-1.76e-05, "Field Reading"=-2.95955946e-05}, {-1.77e-05, "Field Reading"=-2.99420836e-05}, {-1.78e-05, "Field Reading"=-3.00057879e-05}, {-1.79e-05, "Field Reading"=-3.02103666e-05}, {-1.8e-05, "Field Reading"=-3.04377263e-05}, {-1.81e-05, "Field Reading"=-3.058378e-05}, {-1.82e-05, "Field Reading"=-3.06459304e-05}, {-1.83e-05, "Field Reading"=-3.0935966e-05}, {-1.84e-05, "Field Reading"=-3.11265608e-05}, {-1.85e-05, "Field Reading"=-3.14704601e-05}, {-1.86e-05, "Field Reading"=-3.14657988e-05}, {-1.87e-05, "Field Reading"=-3.1490662e-05}, {-1.88e-05, "Field Reading"=-3.16610579e-05}, {-1.89e-05, "Field Reading"=-3.19365917e-05}, {-1.9e-05, "Field Reading"=-3.23074229e-05}, {-1.91e-05, "Field Reading"=-3.24457077e-05}, {-1.92e-05, "Field Reading"=-3.2528575e-05}, {-1.93e-05, "Field Reading"=-3.26357846e-05}, {-1.94e-05, "Field Reading"=-3.27984082e-05}, {-1.95e-05, "Field Reading"=-3.29537844e-05}, {-1.96e-05, "Field Reading"=-3.32728235e-05}, {-1.97e-05, "Field Reading"=-3.33303127e-05}, {-1.98e-05, "Field Reading"=-3.36058465e-05}, {-1.99e-05, "Field Reading"=-3.3674212e-05}, {-2e-05, "Field Reading"=-3.38150864e-05}, {-2.01e-05, "Field Reading"=-3.41139266e-05}, {-2.02e-05, "Field Reading"=-3.43242024e-05}, {-2.03e-05, "Field Reading"=-3.44143206e-05}, {-2.04e-05, "Field Reading"=-3.45091001e-05}, {-2.05e-05, "Field Reading"=-3.46691375e-05}, {-2.06e-05, "Field Reading"=-3.49969813e-05}, {-2.07e-05, "Field Reading"=-3.53066978e-05}, {-2.08e-05, "Field Reading"=-3.53786888e-05}, {-2.09e-05, "Field Reading"=-3.53662716e-05}, {-2.1e-05, "Field Reading"=-3.55413289e-05}, {-2.11e-05, "Field Reading"=-3.57811262e-05}, {-2.12e-05, "Field Reading"=-3.60457838e-05}, {-2.13e-05, "Field Reading"=-3.62638284e-05}, {-2.14e-05, "Field Reading"=-3.6410918e-05}, {-2.15e-05, "Field Reading"=-3.65393623e-05}, {-2.16e-05, "Field Reading"=-3.65880498e-05}, {-2.17e-05, "Field Reading"=-3.68361339e-05}, {-2.18e-05, "Field Reading"=-3.71805513e-05}, {-2.19e-05, "Field Reading"=-3.73499114e-05}, {-2.2e-05, "Field Reading"=-3.73954885e-05}, {-2.21e-05, "Field Reading"=-3.75109848e-05}, {-2.22e-05, "Field Reading"=-3.77254041e-05}, {-2.23e-05, "Field Reading"=-3.80848412e-05}, {-2.24e-05, "Field Reading"=-3.80889931e-05}, {-2.25e-05, "Field Reading"=-3.8286321e-05}, {-2.26e-05, "Field Reading"=-3.8384726e-05}, {-2.27e-05, "Field Reading"=-3.86882277e-05}, {-2.28e-05, "Field Reading"=-3.88389427e-05}, {-2.29e-05, "Field Reading"=-3.90057133e-05}, {-2.3e-05, "Field Reading"=-3.92584588e-05}, {-2.31e-05, "Field Reading"=-3.93149366e-05}, {-2.32e-05, "Field Reading"=-3.93180441e-05}, {-2.33e-05, "Field Reading"=-3.97095927e-05}, {-2.34e-05, "Field Reading"=-3.98862039e-05}, {-2.35e-05, "Field Reading"=-4.01669173e-05}, {-2.36e-05, "Field Reading"=-4.02192274e-05}, {-2.37e-05, "Field Reading"=-4.02497847e-05}, {-2.38e-05, "Field Reading"=-4.05683017e-05}, {-2.39e-05, "Field Reading"=-4.0671368e-05}, {-2.4e-05, "Field Reading"=-4.08997714e-05}, {-2.41e-05, "Field Reading"=-4.11219596e-05}, {-2.42e-05, "Field Reading"=-4.14870942e-05}, {-2.43e-05, "Field Reading"=-4.14062984e-05}, {-2.44e-05, "Field Reading"=-4.14907196e-05}, {-2.45e-05, "Field Reading"=-4.18946983e-05}, {-2.46e-05, "Field Reading"=-4.2003965e-05}, {-2.47e-05, "Field Reading"=-4.21122105e-05}, {-2.48e-05, "Field Reading"=-4.20687051e-05}, {-2.49e-05, "Field Reading"=-4.25596944e-05}, {-2.5e-05, "Field Reading"=-4.26492947e-05}, {-2.51e-05, "Field Reading"=-4.28222804e-05}, {-2.52e-05, "Field Reading"=-4.31263001e-05}, {-2.53e-05, "Field Reading"=-4.31086893e-05}, {-2.54e-05, "Field Reading"=-4.32764958e-05}, {-2.55e-05, "Field Reading"=-4.33593632e-05}, {-2.56e-05, "Field Reading"=-4.37110316e-05}, {-2.57e-05, "Field Reading"=-4.39301122e-05}, {-2.58e-05, "Field Reading"=-4.40041749e-05}, {-2.59e-05, "Field Reading"=-4.41331373e-05}, {-2.6e-05, "Field Reading"=-4.42631313e-05}, {-2.61e-05, "Field Reading"=-4.45738839e-05}, {-2.62e-05, "Field Reading"=-4.49379824e-05}, {-2.63e-05, "Field Reading"=-4.48173068e-05}, {-2.64e-05, "Field Reading"=-4.49369466e-05}, {-2.65e-05, "Field Reading"=-4.50933588e-05}, {-2.66e-05, "Field Reading"=-4.55253049e-05}, {-2.67e-05, "Field Reading"=-4.56335504e-05}, {-2.68e-05, "Field Reading"=-4.56713668e-05}, {-2.69e-05, "Field Reading"=-4.60370191e-05}, {-2.7e-05, "Field Reading"=-4.60225173e-05}, {-2.71e-05, "Field Reading"=-4.62913184e-05}, {-2.72e-05, "Field Reading"=-4.64358184e-05}, {-2.73e-05, "Field Reading"=-4.68377252e-05}, {-2.74e-05, "Field Reading"=-4.70138184e-05}, {-2.75e-05, "Field Reading"=-4.69620301e-05}, {-2.76e-05, "Field Reading"=-4.69578868e-05}, {-2.77e-05, "Field Reading"=-4.72484406e-05}, {-2.78e-05, "Field Reading"=-4.75524603e-05}, {-2.79e-05, "Field Reading"=-4.77751664e-05}, {-2.8e-05, "Field Reading"=-4.77461629e-05}, {-2.81e-05, "Field Reading"=-4.79263994e-05}, {-2.82e-05, "Field Reading"=-4.80688223e-05}, {-2.83e-05, "Field Reading"=-4.83557506e-05}, {-2.84e-05, "Field Reading"=-4.84463868e-05}, {-2.85e-05, "Field Reading"=-4.8701204e-05}, {-2.86e-05, "Field Reading"=-4.88633133e-05}, {-2.87e-05, "Field Reading"=-4.89580929e-05}, {-2.88e-05, "Field Reading"=-4.90720355e-05}, {-2.89e-05, "Field Reading"=-4.94475284e-05}, {-2.9e-05, "Field Reading"=-4.98002004e-05}, {-2.91e-05, "Field Reading"=-4.98701197e-05}, {-2.92e-05, "Field Reading"=-4.98033079e-05}, {-2.93e-05, "Field Reading"=-4.9972668e-05}, {-2.94e-05, "Field Reading"=-5.02689187e-05}, {-2.95e-05, "Field Reading"=-5.0554293e-05}, {-2.96e-05, "Field Reading"=-5.06454471e-05}, {-2.97e-05, "Field Reading"=-5.07350342e-05}, {-2.98e-05, "Field Reading"=-5.09463458e-05}, {-2.99e-05, "Field Reading"=-5.111467e-05}, {-3e-05, "Field Reading"=-5.14104027e-05}, {-3e-05, "Field Reading"=-5.13658615e-05}, {-2.99e-05, "Field Reading"=-5.11198492e-05}, {-2.98e-05, "Field Reading"=-5.10074604e-05}, {-2.97e-05, "Field Reading"=-5.06387154e-05}, {-2.96e-05, "Field Reading"=-5.0536685e-05}, {-2.95e-05, "Field Reading"=-5.0445013e-05}, {-2.94e-05, "Field Reading"=-5.04978409e-05}, {-2.93e-05, "Field Reading"=-5.00317122e-05}, {-2.92e-05, "Field Reading"=-4.99814739e-05}, {-2.91e-05, "Field Reading"=-4.95060226e-05}, {-2.9e-05, "Field Reading"=-4.95572968e-05}, {-2.89e-05, "Field Reading"=-4.95453763e-05}, {-2.88e-05, "Field Reading"=-4.9240321e-05}, {-2.87e-05, "Field Reading"=-4.89280148e-05}, {-2.86e-05, "Field Reading"=-4.87524397e-05}, {-2.85e-05, "Field Reading"=-4.87348304e-05}, {-2.84e-05, "Field Reading"=-4.84815672e-05}, {-2.83e-05, "Field Reading"=-4.84572249e-05}, {-2.82e-05, "Field Reading"=-4.8151152e-05}, {-2.81e-05, "Field Reading"=-4.79351789e-05}, {-2.8e-05, "Field Reading"=-4.78326306e-05}, {-2.79e-05, "Field Reading"=-4.75596863e-05}, {-2.78e-05, "Field Reading"=-4.75659013e-05}, {-2.77e-05, "Field Reading"=-4.71759069e-05}, {-2.76e-05, "Field Reading"=-4.70681794e-05}, {-2.75e-05, "Field Reading"=-4.66564487e-05}, {-2.74e-05, "Field Reading"=-4.6647644e-05}, {-2.73e-05, "Field Reading"=-4.66352139e-05}, {-2.72e-05, "Field Reading"=-4.64290813e-05}, {-2.71e-05, "Field Reading"=-4.608311e-05}, {-2.7e-05, "Field Reading"=-4.59448251e-05}, {-2.69e-05, "Field Reading"=-4.58464201e-05}, {-2.68e-05, "Field Reading"=-4.55724398e-05}, {-2.67e-05, "Field Reading"=-4.55594703e-05}, {-2.66e-05, "Field Reading"=-4.53393539e-05}, {-2.65e-05, "Field Reading"=-4.5103182e-05}, {-2.64e-05, "Field Reading"=-4.49219097e-05}, {-2.63e-05, "Field Reading"=-4.46810766e-05}, {-2.62e-05, "Field Reading"=-4.4776374e-05}, {-2.61e-05, "Field Reading"=-4.44894459e-05}, {-2.6e-05, "Field Reading"=-4.41652463e-05}, {-2.59e-05, "Field Reading"=-4.39544525e-05}, {-2.58e-05, "Field Reading"=-4.39068037e-05}, {-2.57e-05, "Field Reading"=-4.38332589e-05}, {-2.56e-05, "Field Reading"=-4.35779238e-05}, {-2.55e-05, "Field Reading"=-4.33562536e-05}, {-2.54e-05, "Field Reading"=-4.32516335e-05}, {-2.53e-05, "Field Reading"=-4.29408715e-05}, {-2.52e-05, "Field Reading"=-4.27357748e-05}, {-2.51e-05, "Field Reading"=-4.28031045e-05}, {-2.5e-05, "Field Reading"=-4.26342623e-05}, {-2.49e-05, "Field Reading"=-4.25151405e-05}, {-2.48e-05, "Field Reading"=-4.20547087e-05}, {-2.47e-05, "Field Reading"=-4.19423199e-05}, {-2.46e-05, "Field Reading"=-4.18423611e-05}, {-2.45e-05, "Field Reading"=-4.18418278e-05}, {-2.44e-05, "Field Reading"=-4.15678477e-05}, {-2.43e-05, "Field Reading"=-4.11908014e-05}, {-2.42e-05, "Field Reading"=-4.10665004e-05}, {-2.41e-05, "Field Reading"=-4.08070221e-05}, {-2.4e-05, "Field Reading"=-4.07826799e-05}, {-2.39e-05, "Field Reading"=-4.06469846e-05}, {-2.38e-05, "Field Reading"=-4.04175556e-05}, {-2.37e-05, "Field Reading"=-4.02238532e-05}, {-2.36e-05, "Field Reading"=-3.98929018e-05}, {-2.35e-05, "Field Reading"=-3.98970451e-05}, {-2.34e-05, "Field Reading"=-3.9695056e-05}, {-2.33e-05, "Field Reading"=-3.97105936e-05}, {-2.32e-05, "Field Reading"=-3.93449415e-05}, {-2.31e-05, "Field Reading"=-3.90217546e-05}, {-2.3e-05, "Field Reading"=-3.89171346e-05}, {-2.29e-05, "Field Reading"=-3.8966855e-05}, {-2.28e-05, "Field Reading"=-3.87286114e-05}, {-2.27e-05, "Field Reading"=-3.8476384e-05}, {-2.26e-05, "Field Reading"=-3.84276994e-05}, {-2.25e-05, "Field Reading"=-3.80190599e-05}, {-2.24e-05, "Field Reading"=-3.79579453e-05}, {-2.23e-05, "Field Reading"=-3.78610959e-05}, {-2.22e-05, "Field Reading"=-3.77523325e-05}, {-2.21e-05, "Field Reading"=-3.74861212e-05}, {-2.2e-05, "Field Reading"=-3.71494727e-05}, {-2.19e-05, "Field Reading"=-3.71287558e-05}, {-2.18e-05, "Field Reading"=-3.70246537e-05}, {-2.17e-05, "Field Reading"=-3.68356126e-05}, {-2.16e-05, "Field Reading"=-3.65129355e-05}, {-2.15e-05, "Field Reading"=-3.63492726e-05}, {-2.14e-05, "Field Reading"=-3.62058086e-05}, {-2.13e-05, "Field Reading"=-3.59727443e-05}, {-2.12e-05, "Field Reading"=-3.59313107e-05}, {-2.11e-05, "Field Reading"=-3.57930259e-05}, {-2.1e-05, "Field Reading"=-3.55387268e-05}, {-2.09e-05, "Field Reading"=-3.52248795e-05}, {-2.08e-05, "Field Reading"=-3.50436072e-05}, {-2.07e-05, "Field Reading"=-3.51026502e-05}, {-2.06e-05, "Field Reading"=-3.49876718e-05}, {-2.05e-05, "Field Reading"=-3.45391523e-05}, {-2.04e-05, "Field Reading"=-3.44355681e-05}, {-2.03e-05, "Field Reading"=-3.41854124e-05}, {-2.02e-05, "Field Reading"=-3.4246527e-05}, {-2.01e-05, "Field Reading"=-3.40279602e-05}, {-2e-05, "Field Reading"=-3.3930591e-05}, {-1.99e-05, "Field Reading"=-3.36705948e-05}, {-1.98e-05, "Field Reading"=-3.33992043e-05}, {-1.97e-05, "Field Reading"=-3.32324338e-05}, {-1.96e-05, "Field Reading"=-3.32660987e-05}, {-1.95e-05, "Field Reading"=-3.30791293e-05}, {-1.94e-05, "Field Reading"=-3.26730859e-05}, {-1.93e-05, "Field Reading"=-3.25011361e-05}, {-1.92e-05, "Field Reading"=-3.24022132e-05}, {-1.91e-05, "Field Reading"=-3.23203817e-05}, {-1.9e-05, "Field Reading"=-3.21282331e-05}, {-1.89e-05, "Field Reading"=-3.18293927e-05}, {-1.88e-05, "Field Reading"=-3.16978408e-05}, {-1.87e-05, "Field Reading"=-3.13306507e-05}, {-1.86e-05, "Field Reading"=-3.14585772e-05}, {-1.85e-05, "Field Reading"=-3.1275751e-05}, {-1.84e-05, "Field Reading"=-3.10711721e-05}, {-1.83e-05, "Field Reading"=-3.07889051e-05}, {-1.82e-05, "Field Reading"=-3.05651631e-05}, {-1.81e-05, "Field Reading"=-3.05542867e-05}, {-1.8e-05, "Field Reading"=-3.00503494e-05}, {-1.79e-05, "Field Reading"=-3.0249736e-05}, {-1.78e-05, "Field Reading"=-2.99498598e-05}, {-1.77e-05, "Field Reading"=-2.98581878e-05}, {-1.76e-05, "Field Reading"=-2.94101862e-05}, {-1.75e-05, "Field Reading"=-2.94873564e-05}, {-1.74e-05, "Field Reading"=-2.93899872e-05}, {-1.73e-05, "Field Reading"=-2.91703888e-05}, {-1.72e-05, "Field Reading"=-2.89637498e-05}, {-1.71e-05, "Field Reading"=-2.86908053e-05}, {-1.7e-05, "Field Reading"=-2.86628376e-05}, {-1.69e-05, "Field Reading"=-2.83355114e-05}, {-1.68e-05, "Field Reading"=-2.83324038e-05}, {-1.67e-05, "Field Reading"=-2.80734432e-05}, {-1.66e-05, "Field Reading"=-2.78807765e-05}, {-1.65e-05, "Field Reading"=-2.75751979e-05}, {-1.64e-05, "Field Reading"=-2.7529103e-05}, {-1.63e-05, "Field Reading"=-2.76202571e-05}, {-1.62e-05, "Field Reading"=-2.7194526e-05}, {-1.61e-05, "Field Reading"=-2.68361246e-05}, {-1.6e-05, "Field Reading"=-2.67454884e-05}, {-1.59e-05, "Field Reading"=-2.67185565e-05}, {-1.58e-05, "Field Reading"=-2.65424633e-05}, {-1.57e-05, "Field Reading"=-2.63632592e-05}, {-1.56e-05, "Field Reading"=-2.61115496e-05}, {-1.55e-05, "Field Reading"=-2.59297594e-05}, {-1.54e-05, "Field Reading"=-2.57044637e-05}, {-1.53e-05, "Field Reading"=-2.58515533e-05}, {-1.52e-05, "Field Reading"=-2.55392469e-05}, {-1.51e-05, "Field Reading"=-2.53139513e-05}, {-1.5e-05, "Field Reading"=-2.50658771e-05}, {-1.49e-05, "Field Reading"=-2.47121368e-05}, {-1.48e-05, "Field Reading"=-2.49229308e-05}, {-1.47e-05, "Field Reading"=-2.47245669e-05}, {-1.46e-05, "Field Reading"=-2.44469611e-05}, {-1.45e-05, "Field Reading"=-2.4230988e-05}, {-1.44e-05, "Field Reading"=-2.39181635e-05}, {-1.43e-05, "Field Reading"=-2.38798267e-05}, {-1.42e-05, "Field Reading"=-2.38202658e-05}, {-1.41e-05, "Field Reading"=-2.35483573e-05}, {-1.4e-05, "Field Reading"=-2.34805096e-05}, {-1.39e-05, "Field Reading"=-2.32324255e-05}, {-1.38e-05, "Field Reading"=-2.29972894e-05}, {-1.37e-05, "Field Reading"=-2.27502411e-05}, {-1.36e-05, "Field Reading"=-2.26911981e-05}, {-1.35e-05, "Field Reading"=-2.25907217e-05}, {-1.34e-05, "Field Reading"=-2.23819996e-05}, {-1.33e-05, "Field Reading"=-2.2084195e-05}, {-1.32e-05, "Field Reading"=-2.18842775e-05}, {-1.31e-05, "Field Reading"=-2.17926055e-05}, {-1.3e-05, "Field Reading"=-2.17843188e-05}, {-1.29e-05, "Field Reading"=-2.13850017e-05}, {-1.28e-05, "Field Reading"=-2.11141327e-05}, {-1.27e-05, "Field Reading"=-2.1046803e-05}, {-1.26e-05, "Field Reading"=-2.09546131e-05}, {-1.25e-05, "Field Reading"=-2.08075235e-05}, {-1.24e-05, "Field Reading"=-2.05599572e-05}, {-1.23e-05, "Field Reading"=-2.03476095e-05}, {-1.22e-05, "Field Reading"=-2.00891669e-05}, {-1.21e-05, "Field Reading"=-1.99317087e-05}, {-1.2e-05, "Field Reading"=-1.98586819e-05}, {-1.19e-05, "Field Reading"=-1.96913935e-05}, {-1.18e-05, "Field Reading"=-1.95691643e-05}, {-1.17e-05, "Field Reading"=-1.91714012e-05}, {-1.16e-05, "Field Reading"=-1.90175787e-05}, {-1.15e-05, "Field Reading"=-1.89160663e-05}, {-1.14e-05, "Field Reading"=-1.88306093e-05}, {-1.13e-05, "Field Reading"=-1.87197761e-05}, {-1.12e-05, "Field Reading"=-1.83820918e-05}, {-1.11e-05, "Field Reading"=-1.80350849e-05}, {-1.1e-05, "Field Reading"=-1.8132454e-05}, {-1.09e-05, "Field Reading"=-1.78310241e-05}, {-1.08e-05, "Field Reading"=-1.77750886e-05}, {-1.07e-05, "Field Reading"=-1.75938163e-05}, {-1.06e-05, "Field Reading"=-1.72369703e-05}, {-1.05e-05, "Field Reading"=-1.70204794e-05}, {-1.04e-05, "Field Reading"=-1.69578109e-05}, {-1.03e-05, "Field Reading"=-1.67516784e-05}, {-1.02e-05, "Field Reading"=-1.66993684e-05}, {-1.01e-05, "Field Reading"=-1.64968614e-05}, {-1e-05, "Field Reading"=-1.60830426e-05}, {-9.9e-06, "Field Reading"=-1.5979974e-05}, {-9.8e-06, "Field Reading"=-1.59095368e-05}, {-9.7e-06, "Field Reading"=-1.57272287e-05}, {-9.6e-06, "Field Reading"=-1.5542331e-05}, {-9.5e-06, "Field Reading"=-1.53771143e-05}, {-9.4e-06, "Field Reading"=-1.51590697e-05}, {-9.3e-06, "Field Reading"=-1.48804283e-05}, {-9.2e-06, "Field Reading"=-1.48260467e-05}, {-9.1e-06, "Field Reading"=-1.45945374e-05}, {-9e-06, "Field Reading"=-1.4349043e-05}, {-8.9e-06, "Field Reading"=-1.40077331e-05}, {-8.8e-06, "Field Reading"=-1.37855451e-05}, {-8.7e-06, "Field Reading"=-1.40227529e-05}, {-8.6e-06, "Field Reading"=-1.36845506e-05}, {-8.5e-06, "Field Reading"=-1.33551529e-05}, {-8.4e-06, "Field Reading"=-1.32002936e-05}, {-8.3e-06, "Field Reading"=-1.30231648e-05}, {-8.2e-06, "Field Reading"=-1.29547992e-05}, {-8.1e-06, "Field Reading"=-1.27087869e-05}, {-8e-06, "Field Reading"=-1.24881526e-05}, {-7.9e-06, "Field Reading"=-1.2394409e-05}, {-7.8e-06, "Field Reading"=-1.20173627e-05}, {-7.7e-06, "Field Reading"=-1.18744174e-05}, {-7.6e-06, "Field Reading"=-1.15854176e-05}, {-7.5e-06, "Field Reading"=-1.1628923e-05}, {-7.4e-06, "Field Reading"=-1.15051399e-05}, {-7.3e-06, "Field Reading"=-1.09463034e-05}, {-7.2e-06, "Field Reading"=-1.0791963e-05}, {-7.1e-06, "Field Reading"=-1.07505293e-05}, {-7e-06, "Field Reading"=-1.0641248e-05}, {-6.9e-06, "Field Reading"=-1.06241562e-05}, {-6.8e-06, "Field Reading"=-1.03237621e-05}, {-6.7e-06, "Field Reading"=-1.00119739e-05}, {-6.6e-06, "Field Reading"=-9.92133772e-06}, {-6.5e-06, "Field Reading"=-9.80480555e-06}, {-6.4e-06, "Field Reading"=-9.66444903e-06}, {-6.3e-06, "Field Reading"=-9.41066786e-06}, {-6.2e-06, "Field Reading"=-8.84095547e-06}, {-6.1e-06, "Field Reading"=-8.40279443e-06}, {-6e-06, "Field Reading"=-8.10188242e-06}, {-5.9e-06, "Field Reading"=5.24657174e-07}, {-5.8e-06, "Field Reading"=4.10713776e-07}, {-5.7e-06, "Field Reading"=5.03422268e-07}, {-5.6e-06, "Field Reading"=5.80593024e-07}, {-5.5e-06, "Field Reading"=5.74381125e-07}, {-5.4e-06, "Field Reading"=4.99282033e-07}, {-5.3e-06, "Field Reading"=5.10676378e-07}, {-5.2e-06, "Field Reading"=5.8681132e-07}, {-5.1e-06, "Field Reading"=4.81672591e-07}, {-5e-06, "Field Reading"=5.1844525e-07}, {-4.9e-06, "Field Reading"=7.04380243e-07}, {-4.8e-06, "Field Reading"=4.97728259e-07}, {-4.7e-06, "Field Reading"=4.42824878e-07}, {-4.6e-06, "Field Reading"=3.70315445e-07}, {-4.5e-06, "Field Reading"=7.31826761e-07}, {-4.4e-06, "Field Reading"=5.52624877e-07}, {-4.3e-06, "Field Reading"=4.53701293e-07}, {-4.2e-06, "Field Reading"=4.69756953e-07}, {-4.1e-06, "Field Reading"=4.82705066e-07}, {-4e-06, "Field Reading"=5.75413696e-07}, {-3.9e-06, "Field Reading"=6.08560866e-07}, {-3.8e-06, "Field Reading"=5.16888224e-07}, {-3.7e-06, "Field Reading"=5.17924073e-07}, {-3.6e-06, "Field Reading"=3.78084449e-07}, {-3.5e-06, "Field Reading"=5.02386337e-07}, {-3.4e-06, "Field Reading"=6.75373131e-07}, {-3.3e-06, "Field Reading"=6.10631813e-07}, {-3.2e-06, "Field Reading"=3.97764853e-07}, {-3.1e-06, "Field Reading"=4.96688428e-07}, {-3e-06, "Field Reading"=4.80632769e-07}, {-2.9e-06, "Field Reading"=6.17364831e-07}, {-2.8e-06, "Field Reading"=6.11667662e-07}, {-2.7e-06, "Field Reading"=5.23102576e-07}, {-2.6e-06, "Field Reading"=5.53142196e-07}, {-2.5e-06, "Field Reading"=2.34616641e-07}, {-2.4e-06, "Field Reading"=6.30310824e-07}, {-2.3e-06, "Field Reading"=6.30828749e-07}, {-2.2e-06, "Field Reading"=5.43817462e-07}, {-2.1e-06, "Field Reading"=4.5007316e-07}, {-2e-06, "Field Reading"=4.77523149e-07}, {-1.9e-06, "Field Reading"=5.62980662e-07}, {-1.8e-06, "Field Reading"=5.48480248e-07}, {-1.7e-06, "Field Reading"=6.73817961e-07}, {-1.6e-06, "Field Reading"=5.30352893e-07}, {-1.5e-06, "Field Reading"=2.04578426e-07}, {-1.4e-06, "Field Reading"=4.57843473e-07}, {-1.3e-06, "Field Reading"=6.74335885e-07}, {-1.2e-06, "Field Reading"=6.3756325e-07}, {-1.1e-06, "Field Reading"=3.211103e-07}, {-1e-06, "Field Reading"=4.77005528e-07}, {-9e-07, "Field Reading"=4.95650804e-07}, {-8e-07, "Field Reading"=5.0341967e-07}, {-7e-07, "Field Reading"=6.71745082e-07}, {-6e-07, "Field Reading"=5.60909272e-07}, {-5e-07, "Field Reading"=4.17444228e-07}, {-4e-07, "Field Reading"=3.35612182e-07}, {-3e-07, "Field Reading"=4.91508418e-07}, {-2e-07, "Field Reading"=5.73858401e-07}, {-1e-07, "Field Reading"=4.78560308e-07}, {0.0, "Field Reading"=5.23101808e-07}]
  out "data":dbl[](array[numeric])=[5.23101808e-07, 0.0, inf]
  in  "Nanovoltmeter 2182a VISA":refnum<visa-resource-name>="GPIB0::7::INSTR"
  in  "Current source K6221 VISA":refnum<visa-resource-name>="GPIB0::13::INSTR"
  in  "Step":dbl[](array[numeric])=[1e-07, 1e-07, 1e-07] min=-3000.0 max=3000.0 format="%.1e"
  in  "To":dbl[](array[numeric])=[3e-05, -3e-05, 0.0] min=-3000.0 max=3000.0 format="%.1e"
  in  "From":dbl[](array[numeric])=[0.0, 3e-05, -3e-05] min=-3000.0 max=3000.0 format="%.1e"
  in  "file name":string="049_31-05-2022_001_DevB4_DC_IV_I_10-36_V_12-37_100nA_steps_baseT_ZFC_afterwarmup"
  out "File path":path=path "D:/Pranava/Data/PtTe2/31-05-2022/001/Round8_IP/after warmup/049_31-05-2022_001_DevB4_DC_IV_I_10-36_V_12-37_100nA_steps_baseT_ZFC_afterwarmup.dat"
  # ".dat"
  # "Set Current (A)"
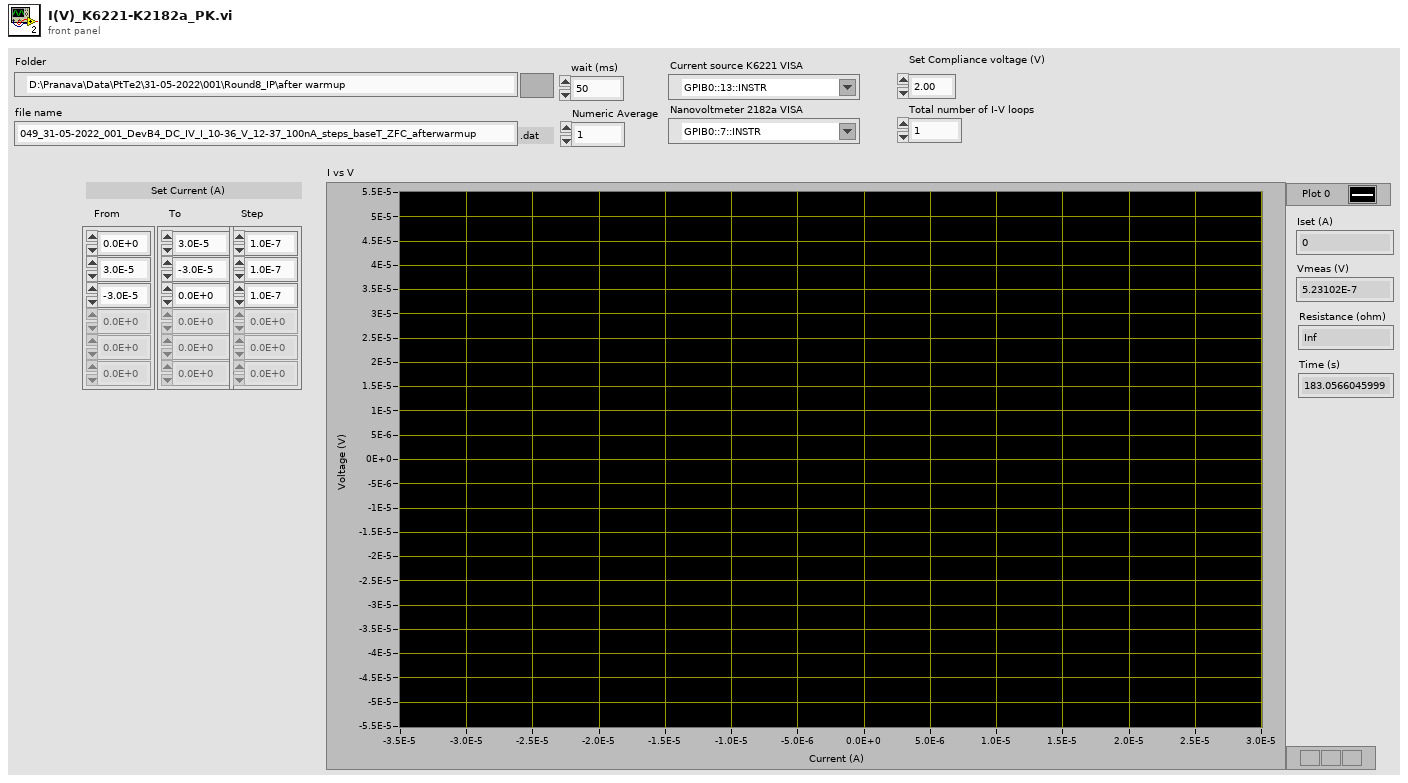
[diagram p1: front panel]
types:
  T1 = enum16{"open", "replace", "create", "open or create", "replace or create", "replace or create with confirmation"}
  T2 = typedef "Keithley 622x.lvlib/KE622x -- Current Level.ctl" = dbl
  T3 = cluster{"Average value":dbl, "Average value":dbl}
  T4 = cluster{"Average value":dbl, "Average value":dbl}[]
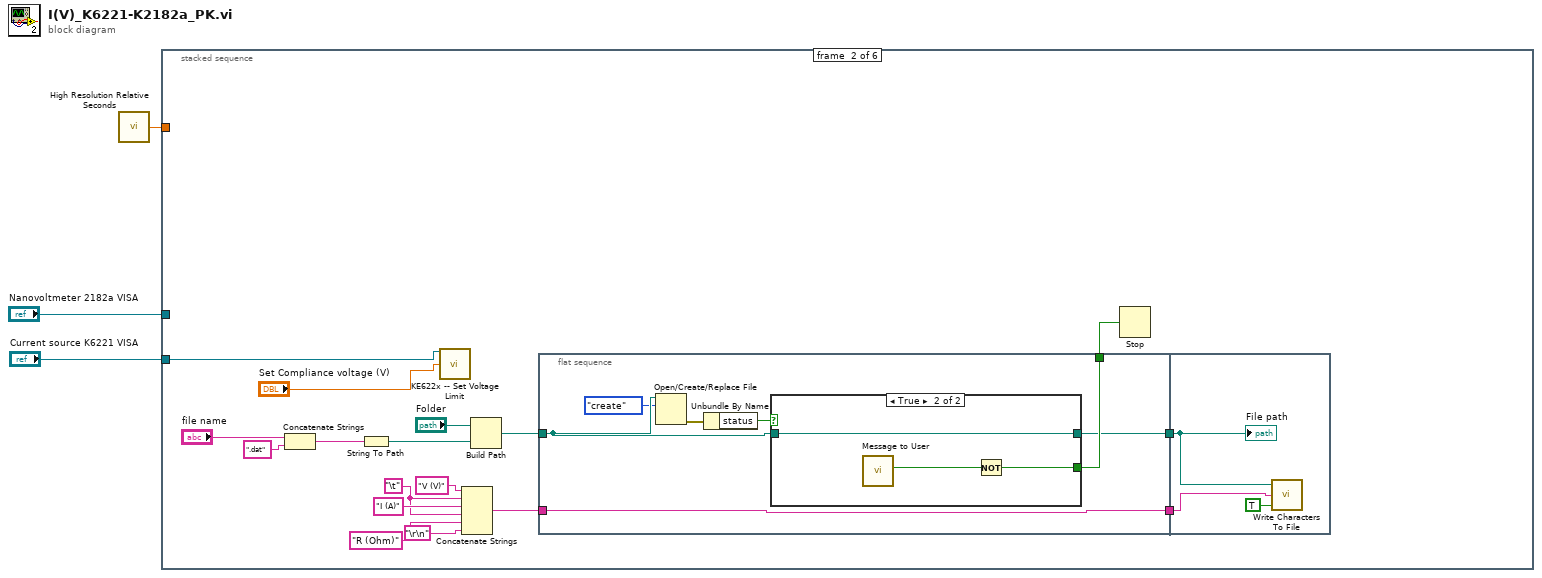
[diagram p0: block diagram]
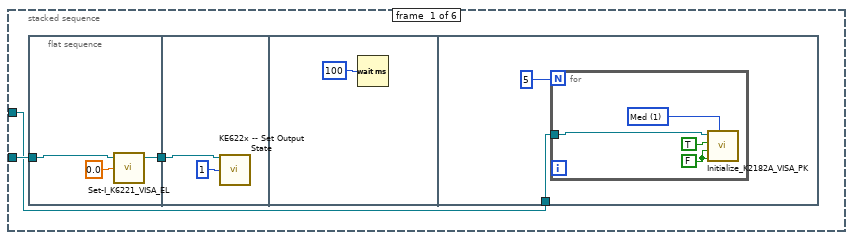
[diagram p2: hidden frame]
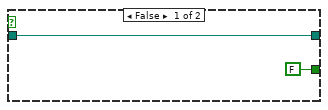
[diagram p3: hidden frame]
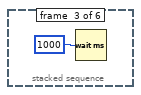
[diagram p4: hidden frame]
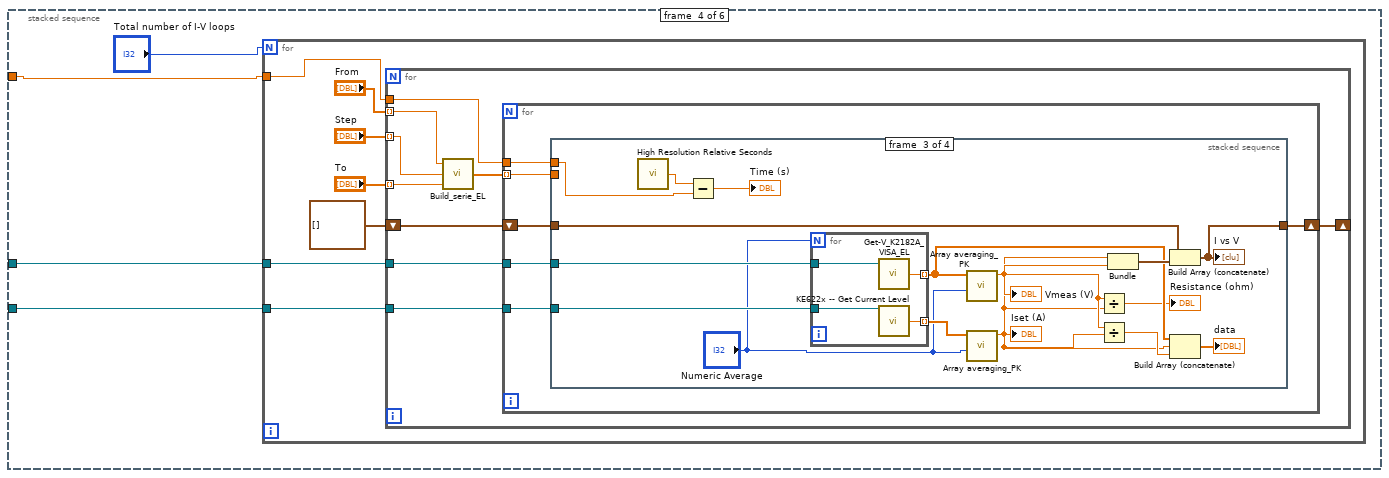
[diagram p5: hidden frame]
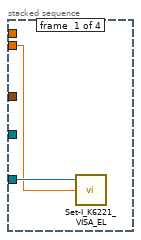
[diagram p6: hidden frame]
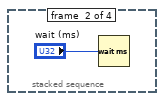
[diagram p7: hidden frame]
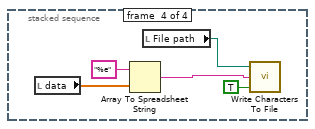
[diagram p8: hidden frame]
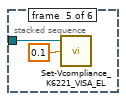
[diagram p9: hidden frame]
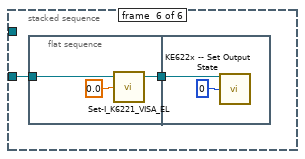
[diagram p10: hidden frame]
diagram:
  n1 = call <vilib>:"High Resolution Relative Seconds.vi"() -> ("relative seconds"=w1:dbl)
  n2 = stacked-sequence {
    tunnel: "Nanovoltmeter 2182a VISA" -> [w4 _ _ w55 _ _]
    tunnel: "Current source K6221 VISA" -> [w5 w20 _ w54 w107 w109]
    tunnel: w1 -> [_ _ _ w52 _ _]
    frame #0 {
      n3 = flat-sequence {
        tunnel: w5 -> [w9]
        tunnel: [w7] -> w6
        tunnel: w6 -> [w11]
        tunnel: w4 -> [w13]
        frame #0 {
          n4 = call "Set-I_K6221_VISA_EL.vi"("Set I (A)"=0.0, "K6221 VISA"=w9) -> ("K6221 VISA out"=w7:refnum<visa-resource-name>)  [unwired: 2 in, 1 out]
        }
        frame #1 {
          n5 = call "KE622x -- Set Output State.vi"("Resource In"=w11, "Output State"=1) -> ()  [unwired: 12 in, 2 out]
        }
        frame #2 {
          n6 = Wait (ms)(milliseconds to wait=100) -> ()  [unwired: 1 out]
        }
        frame #3 {
          n7 = for {
            N: 5 ("Numeric") -> [_]
            tunnel: w13 -> [w15]
            w17 = u16 1 items=["Slow", "Med", "Fast"] ("Rate (NPLC)")
            w18 = FALSE ("Auto range?")
            n8 = call "Initialize_K2182A_VISA_PK.vi"("VISA address"=w15, "Auto range?"=TRUE, "Analog LPass\nFilter?"=w18, "DC\nFilter?"=w18, "Rate (NPLC)"=w17) -> ()  [unwired: 2 in]
          }
        }
      }
    }
    frame #1 {
      w26 = "\t"
      n9 = Concatenate Strings("file name", ".dat" ("string")) -> (w32:string)
      n10 = String To Path(string=w32) -> (path=w22:path)
      n11 = call "KE622x -- Set Voltage Limit.vi"("Resource In"=w20, "Voltage Limit (V)"="Set Compliance voltage (V)") -> ()  [unwired: 12 in, 2 out]
      n12 = Concatenate Strings("V (V)" ("string"), w26, "I (A)" ("string"), w26, "R (Ohm)" ("string"), "\r\n") -> (w33:string)
      n13 = Build Path(base path="Folder", name or relative path=w22) -> (appended path=w21:path)
      n14 = flat-sequence {
        tunnel: w21 -> [w39]
        tunnel: w33 -> [w42]
        tunnel: [w42] -> w35
        tunnel: [w41] -> w30
        tunnel: [w40] -> w34
        tunnel: w35 -> [w49]
        tunnel: w34 -> [w48]
        frame #0 {
          n15 = Open/Create/Replace File(file path (use dialog)=w39, operation (0:open)=T1."create") -> (error out=w38:errorcluster)  [unwired: 4 in, 2 out]
          n16 = Unbundle By Name(w38) -> ("status"=w36:bool)
          n17 = case shown="True" w36 {
            tunnel: [FALSE ("Yes") w46] -> w41
            tunnel: [w43 w45] -> w40
            tunnel: w39 -> [w43 w45]
            frame False {
            }
            frame True {
              n18 = call "Message to User"() -> ("Yes"=w47:bool)  [unwired: 10 in, 1 out]
              n19 = Not(x=w47) -> (.not. x?=w46:bool)
            }
          }
        }
        frame #1 {
          n20 = call <vilib>:"Write Characters To File.vi"("append to file? (new file:F)"=TRUE, "character string"=w49, "file path (dialog if empty)"=w48) -> ()  [unwired: 2 in, 1 out]
          "File path" <- w48
        }
      }
      n21 = Stop(stop? (T)=w30) -> ()
    }
    frame #2 {
      n22 = Wait (ms)(milliseconds to wait=u32 1000) -> ()  [unwired: 1 out]
    }
    frame #3 {
      n23 = for {
        N: "Total number of I-V loops" -> [_]
        tunnel: w55 -> [w59]
        tunnel: w54 -> [w58]
        tunnel: w52 -> [w56]
        n24 = for {
          tunnel: "From" -> [w66] mode=indexing
          tunnel: "To" -> [w65] mode=indexing
          tunnel: "Step" -> [w64] mode=indexing
          tunnel: w59 -> [w71]
          tunnel: w58 -> [w70]
          shift-right: [w68] -> _
          shift-left: cluster{dbl, "Field Reading":dbl}[] [] -> [w69]
          tunnel: w56 -> [w63]
          n25 = call "Build_serie_EL.vi"("end value"=w65, "increment"=w64, "start value"=w66) -> ("output array"=w67:dbl[])
          n26 = for {
            tunnel: w67 -> [w75] mode=indexing
            tunnel: w71 -> [w77]
            tunnel: w70 -> [w76]
            shift-right: [w73] -> w68
            shift-left: w69 -> [w74]
            tunnel: w63 -> [w72]
            n27 = stacked-sequence {
              tunnel: w77 -> [_ _ w91 _]
              tunnel: w76 -> [w79 _ w90 _]
              tunnel: w74 -> [_ _ w94 _]
              tunnel: w75 -> [w78 _ _ _]
              tunnel: [_ _ w93 _] -> w73
              tunnel: w72 -> [_ _ w83 _]
              frame #0 {
                n28 = call "Set-I_K6221_VISA_EL.vi"("Set I (A)"=w78, "K6221 VISA"=w79) -> ()  [unwired: 2 in, 2 out]
              }
              frame #1 {
                n29 = Wait (ms)(milliseconds to wait="wait (ms)") -> ()  [unwired: 1 out]
              }
              frame #2 {
                n30 = call <vilib>:"High Resolution Relative Seconds.vi"() -> ("relative seconds"=w82:dbl)
                n31 = Subtract(x=w82, y=w83) -> (x-y=→"Time (s)":dbl)
                n32 = for {
                  N: "Numeric Average" -> [_]
                  tunnel: [w100] -> w92 mode=indexing
                  tunnel: w91 -> [w99]
                  tunnel: w90 -> [w98]
                  tunnel: [w97] -> w89 mode=indexing
                  n33 = call "Get-V_K2182A_VISA_EL.vi"("VISA K2182A"=w99) -> ("V (V)"=w100:dbl)  [unwired: 2 in, 2 out]
                  n34 = call "KE622x -- Get Current Level.vi"("Resource In"=w98) -> ("Current Level (A)"=w97:T2)  [unwired: 12 in, 2 out]
                }
                n35 = call "Array averaging_PK.vi"("Number averaging"="Numeric Average", "numeric array"=w92) -> ("Average value"=w86:dbl)  [unwired: 9 in]
                "Vmeas (V)" <- w86
                n36 = call "Array averaging_PK.vi"("Number averaging"="Numeric Average", "numeric array"=w89) -> ("Average value"=w85:dbl)  [unwired: 9 in]
                "Iset (A)" <- w85
                n37 = Divide(x=w86, y=w85) -> (x/y=→"Resistance (ohm)":dbl)
                n38 = Divide(x=w86, y=w85) -> (x/y=w87:dbl)
                n39 = Bundle("Average value"=w85, "Average value"=w86) -> (w95:T3)  [unwired: 1 in]
                n40 = Build Array (concatenate)(w94, w95) -> (w93:T4)
                "I vs V" <- w93
                n41 = Build Array (concatenate)(w92, w85, w87) -> (→"data":dbl[])
              }
              frame #3 {
                n42 = local read "data"() -> (w101:dbl[])
                n43 = Array To Spreadsheet String(array=w101, 3:"%e" ("format string")) -> (spreadsheet string=w104:string)  [unwired: 1 in]
                n44 = local read "File path"() -> (w103:path)
                n45 = call <vilib>:"Write Characters To File.vi"("append to file? (new file:F)"=TRUE, "character string"=w104, "file path (dialog if empty)"=w103) -> ()  [unwired: 2 in, 1 out]
              }
            }
          }
        }
      }
    }
    frame #4 {
      n46 = call "Set-Vcompliance_K6221_VISA_EL.vi"("Set Compliance voltage (V)"=0.1, "K6221 VISA"=w107) -> ()  [unwired: 2 in, 2 out]
    }
    frame #5 {
      n47 = flat-sequence {
        tunnel: w109 -> [w112]
        tunnel: [w110] -> w108
        tunnel: w108 -> [w114]
        frame #0 {
          n48 = call "Set-I_K6221_VISA_EL.vi"("Set I (A)"=0.0, "K6221 VISA"=w112) -> ("K6221 VISA out"=w110:refnum<visa-resource-name>)  [unwired: 2 in, 1 out]
        }
        frame #1 {
          n49 = call "KE622x -- Set Output State.vi"("Resource In"=w114, "Output State"=0) -> ()  [unwired: 12 in, 2 out]
        }
      }
    }
  }
